vi "Get States for Motion Trigger.vi"(8 "error in (no error)":errorcluster, 9 "Names only?":bool, 10 "old Motor States in":T1, 11 "new Motor States in":T1) -> (0 "error out":errorcluster, 1 "Array of Trigger State Names":string[](array[string])=["True", "False", "Move Complete", "Motion Incomplete"], 2 "States LUT (name -> boolean state)":variant, 3 "new Motor States out":T1)   [LabVIEW 2016, in "Hardware.lvlib" / "Motions.lvlib" / "Motions.lvclass"]
uses:
  <userlib>/Common Components/Hardware/Abstract System/Motions/Motions/Motions.lvclass
  <userlib>/Common Components/Hardware/Abstract System/Motions/Motions/Motor States.ctl
  <userlib>/Common Components/TriggerAction Q/TriggerAction Q/TriggerAction Q.lvclass
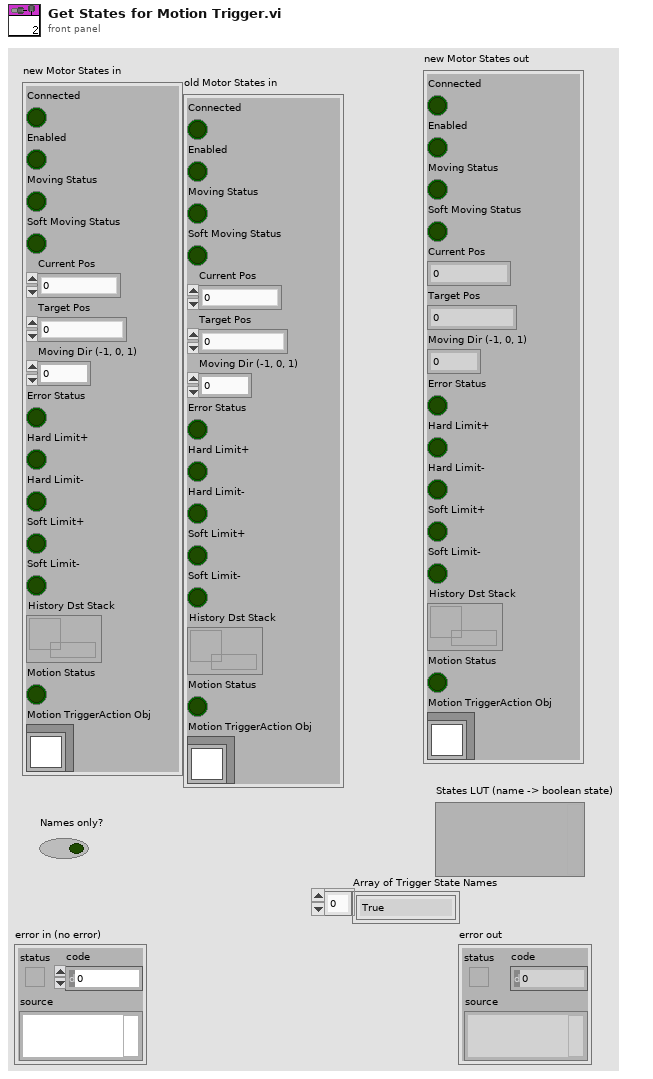
[diagram p1: front panel]
types:
  T1 = typedef "Hardware.lvlib/Motions.lvlib/Motions.lvclass/Motor States.ctl" = cluster{"Connected":bool, "Enabled":bool, "Moving Status":bool, "Soft Moving Status":bool, "Current Pos":dbl, "Target Pos":dbl, "Moving Dir (-1, 0, 1)":i32, "Error Status":bool, "Hard Limit+":bool, "Hard Limit-":bool, "Soft Limit+":bool, "Soft Limit-":bool, "History Dst Stack":refnum<queue>, "Motion Status":bool, "Motion TriggerAction Obj":refnum<class "TriggerAction Q.lvclass">}
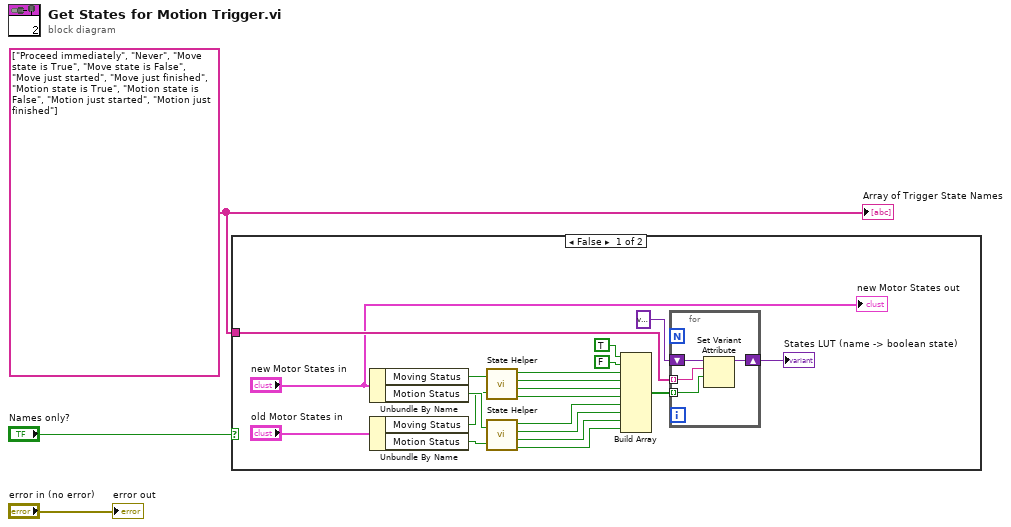
[diagram p0: block diagram]
diagram:
  w2 = string[] ["Proceed immediately", "Never", "Move state is True", "Move state is False", "Move just started", "Move just finished", "Motion state is True", "Motion state is False", "Motion just started", "Motion just finished"] ("Array of Trigger State Names")
  n1 = case shown="False" "Names only?" {
    tunnel: w2 -> [w22 _]
    frame False {
      n2 = Unbundle By Name("new Motor States in") -> ("Moving Status"=w15:bool, "Motion Status"=w14:bool)
      n3 = Unbundle By Name("old Motor States in") -> ("Moving Status"=w13:bool, "Motion Status"=w12:bool)
      n4 = call <userlib>:"State Helper.vi"("new state"=w15, "old state"=w13) -> ("new state is True?"=w11:bool, "new state is False?"=w10:bool, "new state changed to True?"=w9:bool, "new state changed to False?"=w8:bool)
      n5 = call <userlib>:"State Helper.vi"("new state"=w14, "old state"=w12) -> ("new state is True?"=w7:bool, "new state is False?"=w6:bool, "new state changed to True?"=w5:bool, "new state changed to False?"=w4:bool)
      n6 = Build Array(TRUE, FALSE, w11, w10, w9, w8, w7, w6, w5, w4) -> (w20:bool[])
      n7 = for {
        shift-right: [w26] -> w21
        shift-left: variant -> [w27]
        tunnel: w22 -> [w25] mode=indexing
        tunnel: w20 -> [w24] mode=indexing
        n8 = Set Variant Attribute(Variant=w27, name=w25, value=w24) -> (Variant out=w26:variant)  [unwired: 1 in, 2 out]
      }
      "States LUT (name -> boolean state)" <- w21
      "new Motor States out" <- "new Motor States in"
    }
    frame True {
    }
  }
  "error out" <- "error in (no error)"
  "Array of Trigger State Names" <- w2
